vi "Get Device Information.vi"(8 "error in":errorcluster, 10 "RIO Target in":refnum<class "RIO Target.lvclass">, 11 "Bus in":refnum<class "Bus.lvclass">) -> (0 "error out":errorcluster, 1 "Enable Lines":string[](array[string]), 2 "Chip Select Lines":string[](array[string]), 3 "Bus out":refnum<class "Bus.lvclass">, 5 "Device Information Array":T1[](array[typedef]))   [LabVIEW 2014, in "Bus.lvclass"]
uses:
  Bus.lvclass
  Scripting/Initialization Scripting/State Machine/Controls/Device Information.ctl
  RIO Target/RIO Target.lvclass
  <vilib>/NI/Configuration Framework/Node/NISE_CEF_Node.lvclass/NISE_CEF_Node.ctl
  Device node/Device.lvclass
  Device Configuration/Device Configuration.lvclass
  Device Configuration/Device Configuration.lvclass/Device Configuration.ctl
  <vilib>/NI/Configuration Framework/serializable configuration/read metadata property.vi
  <vilib>/NI/Configuration Framework/Node/NISE_CEF_Node.lvclass
  <vilib>/NI/Configuration Framework/serializable configuration/NISE_CEF_serializable configuration.lvclass
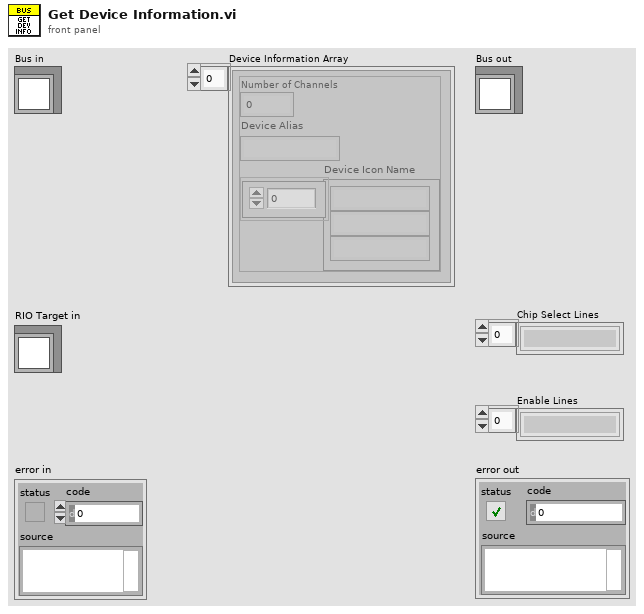
[diagram p1: front panel]
types:
  T1 = typedef "Device Information.ctl" = cluster{"Number of Channels":i32, "Device Alias":string, "Device Icon Name":string[]}
  T2 = typedef "NISE_CEF_Node.lvclass/NodeRef.ctl" = refnum<data-value>
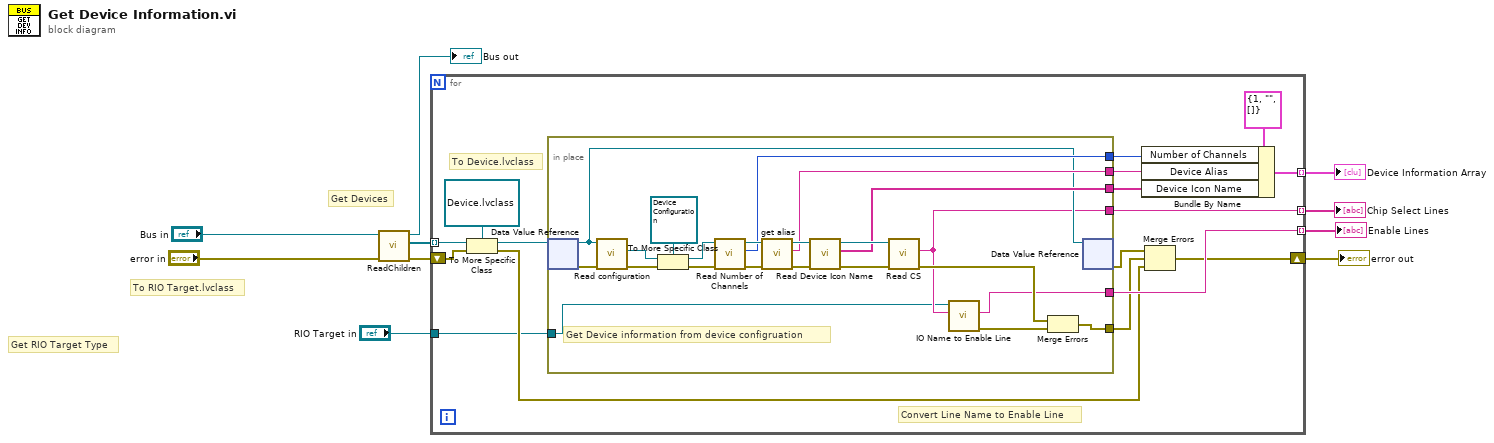
[diagram p0: block diagram]
diagram:
  # "Get RIO Target Type"
  # "To RIO Target.lvclass"
  # "Get Devices"
  n1 = call <vilib>:"ReadChildren.vi"("error in"="error in", "node in"="Bus in") -> ("error out"=w10:errorcluster, "output array"=w8:T2[], "node out"=→"Bus out":refnum<class "Bus.lvclass">)  [unwired: 7 in]
  n2 = for {
    tunnel: w8 -> [w26] mode=indexing
    tunnel: [w22] -> w9 mode=indexing
    shift-right: [w15] -> w5
    shift-left: w10 -> [w21]
    tunnel: [w17] -> w6 mode=indexing
    tunnel: [w12] -> w4 mode=indexing
    tunnel: "RIO Target in" -> [w11]
    # "Convert Line Name to Enable Line"
    # "To Device.lvclass"
    n3 = To More Specific Class(target class=refnum<data-value> refnum ("data value reference"), reference=w26, error in=w21) -> (specific class reference=w24:refnum<data-value>, error out=w13:errorcluster)
    n4 = in-place {
      in-place-border: [w34] -> w17
      in-place-border: [w33] -> w14
      in-place-border: [w32] -> w20
      in-place-border: [w31] -> w19
      in-place-border: [w30] -> w18
      in-place-border: [w28] -> w12
      in-place-border: w11 -> [w27]
      # "Get Device information from device configruation"
      n5 = in-place-dvr #1(w24) -> (w29:refnum<class "Device.lvclass">, w45:errorcluster)
      n6 = call-dynamic "Read configuration.vi"("error in"=w45, "Device in"=w29) -> ("error out"=w44:errorcluster, "configuration"=w48:refnum<class "NISE_CEF_serializable configuration.lvclass">)  [unwired: 7 in, 1 out]
      n7 = To More Specific Class(target class=refnum<class "Device Configuration.lvclass"> refnum ("Device Configuration.lvclass"), reference=w48, error in=w44) -> (specific class reference=w46:refnum<class "Device Configuration.lvclass">, error out=w43:errorcluster)
      n8 = call "Read Number of Channels.vi"("error in (no error)"=w43, "Device Configuration in"=w46) -> ("error out"=w39:errorcluster, "Number of Channels"=w32:u32, "Device Configuration out"=w40:refnum<class "Device Configuration.lvclass">)  [unwired: 7 in]
      n9 = call <vilib>:"get alias.vi"("error in"=w39, "configuration in"=w40) -> ("error out"=w41:errorcluster, "alias"=w31:string, "configuration out"=w42:refnum<class "Device Configuration.lvclass">)  [unwired: 7 in]
      n10 = call "Read Device Icon Name.vi"("error in (no error)"=w41, "Device Configuration in"=w42) -> ("error out"=w37:errorcluster, "Device Icon Name"=w30:string[], "Device Configuration out"=w38:refnum<class "Device Configuration.lvclass">)  [unwired: 7 in]
      n11 = call "Read CS.vi"("error in (no error)"=w37, "Device Configuration in"=w38) -> ("error out"=w36:errorcluster, "CS"=w28:string)  [unwired: 7 in, 1 out]
      n12 = call-dynamic "IO Name to Enable Line.vi"("IO Name"=w28, "RIO Target in"=w27) -> ("error out"=w35:errorcluster, "Enable Line"=w34:string)  [unwired: 7 in, 1 out]
      n13 = Merge Errors(w36, w35) -> (w33:errorcluster)
      n14 = in-place-dvr #1(w29) -> (w16:errorcluster)  [unwired: 1 out]
    }
    n15 = Bundle By Name(cluster=T1 {"Number of Channels"=1, "Device Alias"="", "Device Icon Name"=[]} ("Device Information"), "Number of Channels"=w20, "Device Alias"=w19, "Device Icon Name"=w18) -> (w22:T1)
    n16 = Merge Errors(w16, w14, w13) -> (w15:errorcluster)
  }
  "Device Information Array" <- w9
  "Enable Lines" <- w6
  "error out" <- w5
  "Chip Select Lines" <- w4
